vi "Process Message.vi"(8 "error in (no error)":errorcluster, 9 "Error From Read":errorcluster, 10 "Message":string, 11 "tWorkerTCPConnection in":refnum<class "tWorkerTCPConnection.lvclass">) -> (0 "error out":errorcluster, 3 "tWorkerTCPConnection out":refnum<class "tWorkerTCPConnection.lvclass">)   [LabVIEW 2014, in "tWorkerTCPConnection.lvlib" / "tWorkerTCPConnection.lvclass"]
uses:
  tWorkerTCPConnection.lvclass
  tWorkerTCPConnection.lvclass/tWorkerTCPConnection.ctl
  tWorkerCommandRunner/msgs/Run VI Msg/Run VI.lvclass/Run VI.ctl
  <vilib>/ActorFramework/Message Enqueuer/Message Enqueuer.lvclass/Message Enqueuer.ctl
  BSON/tBSONDocument/tBSONDocument.lvclass
  <vilib>/ActorFramework/Actor/Actor.lvclass/Actor.ctl
  tWorkerController/msgs/TCP Connection Lost Msg/TCP Connection Lost Msg.lvclass/TCP Connection Lost Msg.ctl
  <vilib>/ActorFramework/Message Enqueuer/Enqueue.vi
  <vilib>/ActorFramework/Message Enqueuer/Init from Existing Queue.vi
  BSON/tBSONDocument/getStringValue.vi
  BSON/tBSONDocument/getI32Value.vi
  BSON/tBSONDocument/getBooleanValue.vi
  BSON/tBSONDocument/getString[]Value.vi
  BSON/tBSONDocument/getDocumentValue.vi
  <vilib>/ActorFramework/Message Priority Queue/Priority Enqueue.vi
  tWorkerCommandRunner/msgs/Run VI Msg/Run VI.lvclass
  <vilib>/ActorFramework/Message Enqueuer/Message Enqueuer.lvclass
  tWorkerController/msgs/TCP Connection Lost Msg/TCP Connection Lost Msg.lvclass
  <vilib>/ActorFramework/Stop Msg/Stop Msg.lvclass
  <vilib>/ActorFramework/Actor/Actor.lvclass
  tWorkerController/msgs/TCP Command Received Msg/TCP Command Received Msg.lvclass
  tWorkerCommandRunner/msgs/Describe Error Msg/Describe Error Msg.lvclass
  tWorkerCommandRunner/msgs/Set Controls Msg/Set Controls.lvclass
  tWorkerCommandRunner/msgs/Get Indicators Msg/Get Indicators.lvclass
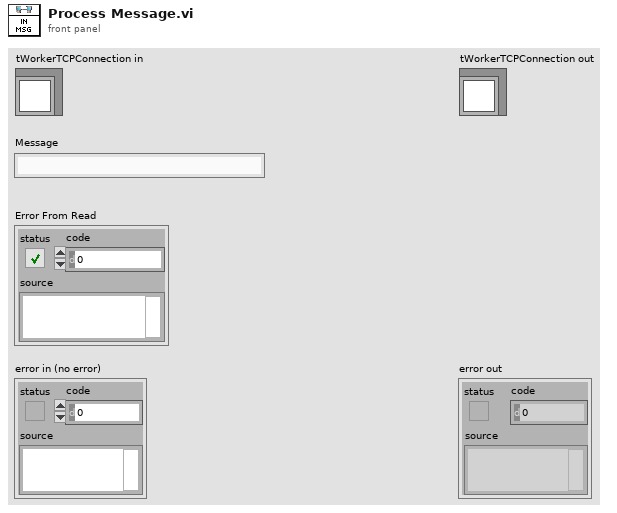
[diagram p1: front panel]
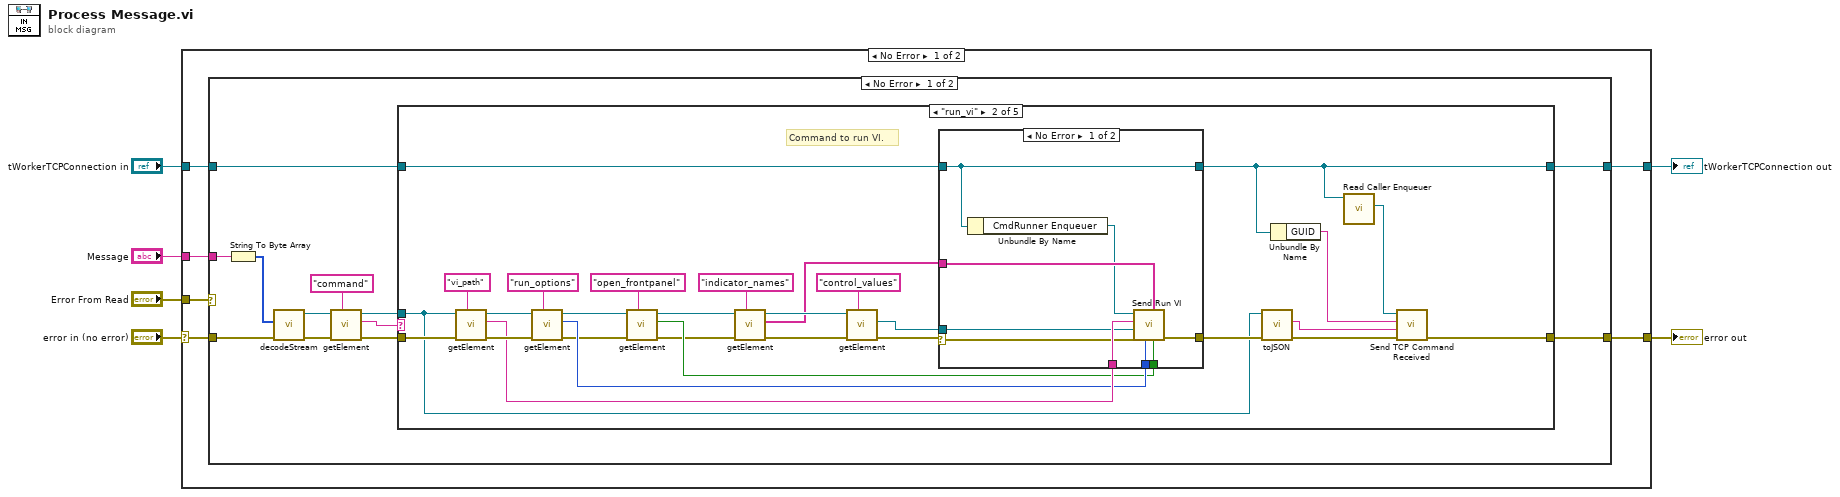
[diagram p0: block diagram]
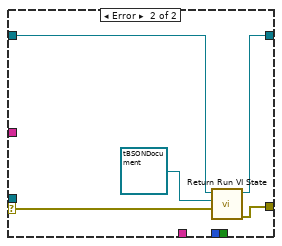
[diagram p3: hidden frame]
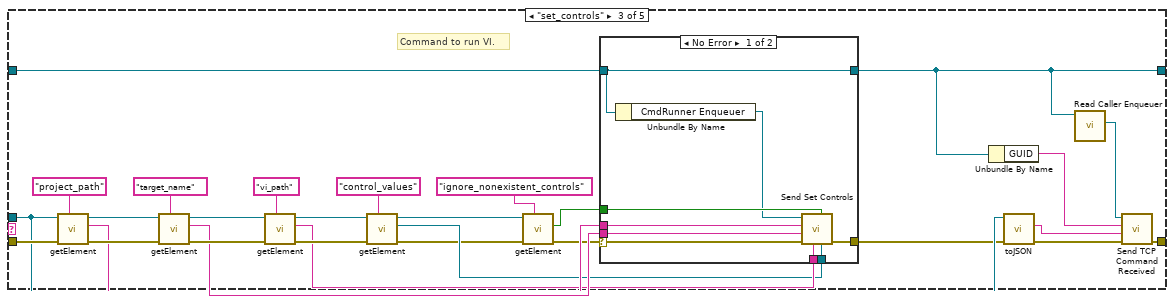
[diagram p4: hidden frame]
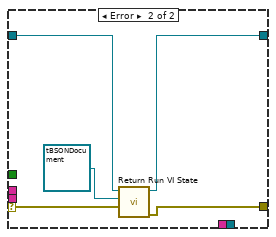
[diagram p5: hidden frame]
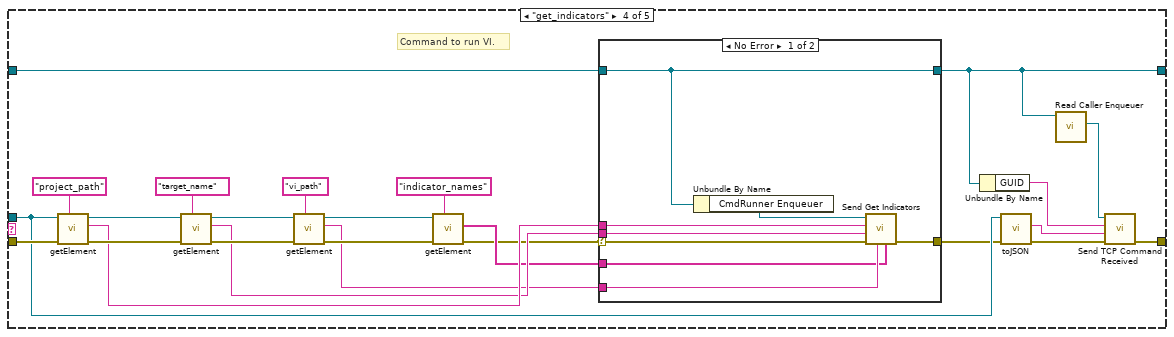
[diagram p6: hidden frame]
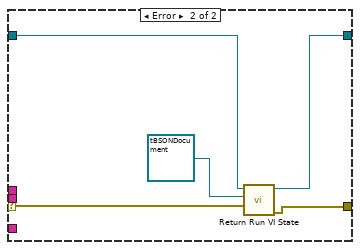
[diagram p7: hidden frame]
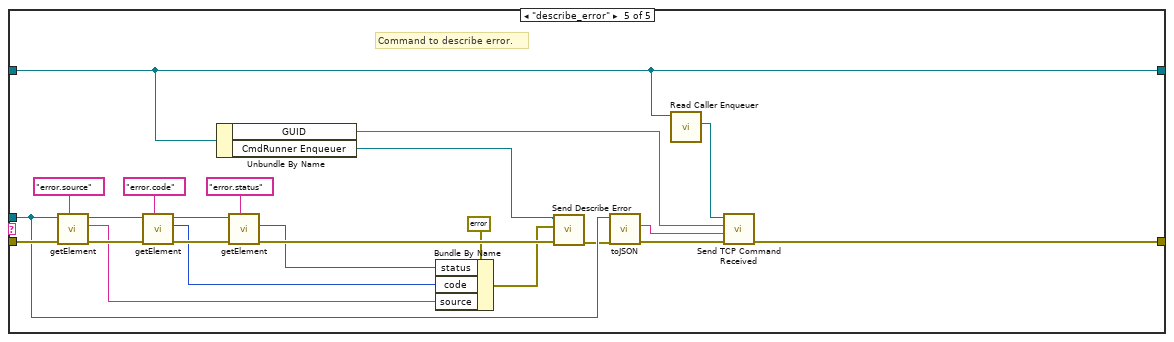
[diagram p8: hidden frame]
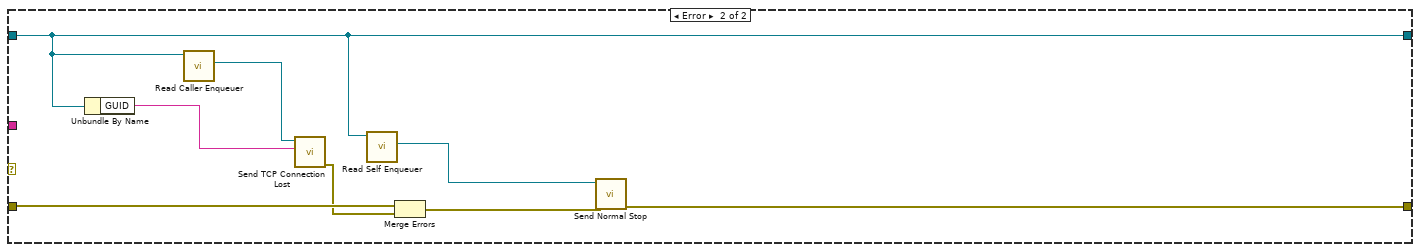
[diagram p9: hidden frame]
diagram:
  n1 = case shown="No Error" "error in (no error)" {
    selector: "error in (no error)" -> [w10 w183]
    tunnel: [w7 w183] -> w5
    tunnel: [w8 w182] -> w3
    tunnel: "tWorkerTCPConnection in" -> [w12 w182]
    tunnel: "Message" -> [w11 _]
    tunnel: "Error From Read" -> [w9 _]
    frame No Error {
      n2 = case shown="No Error" w9 {
        tunnel: w12 -> [w24 w174]
        tunnel: w11 -> [w22 _]
        tunnel: w10 -> [w23 w179]
        tunnel: [w20 w174] -> w8
        tunnel: [w19 w176] -> w7
        frame No Error {
          n3 = String To Byte Array(string=w22) -> (unsigned byte array=w21:u8[])
          n4 = call "decodeStream.vi"("error in (no error)"=w23, "Byte Data In"=w21) -> ("error out"=w17:errorcluster, "tBSONDocument out"=w18:refnum<class "tBSONDocument.lvclass">)  [unwired: 6 in, 2 out]
          n5 = call-poly "getElement.vi"("Name"="command", "error in (no error)"=w17, "tBSONDocument in"=w18) -> ("error out"=w15:errorcluster, "Value"=w13:string, "tBSONDocument out"=w16:refnum<class "tBSONDocument.lvclass">)  [unwired: 6 in]
          n6 = case shown="\"run_vi\"" w13 {
            tunnel: w24 -> [w25 w29 w72 w116 w168]
            tunnel: w16 -> [_ w42 w89 w128 w163]
            tunnel: w15 -> [w26 w50 w93 w132 w169]
            tunnel: [w25 w28 w71 w113 w168] -> w20
            tunnel: [w26 w46 w92 w131 w167] -> w19
            frame Default {
              # "Invalid Command"
            }
            frame "run_vi" {
              # "Command to run VI."
              n7 = call-poly "getElement.vi"("Name"="vi_path", "error in (no error)"=w50, "tBSONDocument in"=w42) -> ("error out"=w55:errorcluster, "Value"=w49:string, "tBSONDocument out"=w54:refnum<class "tBSONDocument.lvclass">)  [unwired: 6 in]
              n8 = call-poly "getElement.vi"("Name"="run_options", "error in (no error)"=w55, "tBSONDocument in"=w54) -> ("error out"=w40:errorcluster, "Value"=w47:i32, "tBSONDocument out"=w39:refnum<class "tBSONDocument.lvclass">)  [unwired: 6 in]
              n9 = call-poly "getElement.vi"("Name"="open_frontpanel", "error in (no error)"=w40, "tBSONDocument in"=w39) -> ("error out"=w34:errorcluster, "Value"=w37:bool, "tBSONDocument out"=w35:refnum<class "tBSONDocument.lvclass">)  [unwired: 6 in]
              n10 = call-poly "getElement.vi"("Name"="indicator_names", "error in (no error)"=w34, "tBSONDocument in"=w35) -> ("error out"=w32:errorcluster, "Value"=w31:string[], "tBSONDocument out"=w33:refnum<class "tBSONDocument.lvclass">)  [unwired: 6 in]
              n11 = call-poly "getElement.vi"("Name"="control_values", "error in (no error)"=w32, "tBSONDocument in"=w33) -> ("error out"=w30:errorcluster, "Value"=w48:refnum<class "tBSONDocument.lvclass">)  [unwired: 6 in, 1 out]
              n12 = case shown="No Error" w30 {
                selector: w30 -> [w58 w69]
                tunnel: w49 -> [w64 _]
                tunnel: w48 -> [w63 _]
                tunnel: w47 -> [w62 _]
                tunnel: [w61 w66] -> w44
                tunnel: w37 -> [w60 _]
                tunnel: w31 -> [w59 _]
                tunnel: w29 -> [w57 w68]
                tunnel: [w57 w67] -> w28
                frame No Error {
                  n13 = Unbundle By Name(w57) -> ("CmdRunner Enqueuer"=w56:refnum<class "Message Enqueuer.lvclass">)
                  n14 = call "Send Run VI.vi"("Open Front Panel"=w60, "Indicator Names"=w59, "Run Options"=w62, "error in (no error)"=w58, "VI Control Values"=w63, "VI Path"=w64, "Message Enqueuer"=w56) -> ("error out"=w61:errorcluster)  [unwired: 3 in, 1 out]
                }
                frame Error {
                  n15 = call "Return Run VI State.vi"("Error From Run VI"=w69, "Indicators"=refnum<class "tBSONDocument.lvclass"> refnum, "tWorkerTCPConnection in"=w68) -> ("error out"=w66:errorcluster, "tWorkerTCPConnection out"=w67:refnum<class "tWorkerTCPConnection.lvclass">)  [unwired: 7 in]
                }
              }
              n16 = call-dynamic "toJSON.vi"("error in (no error)"=w44, "tBSONDocument in"=w42) -> ("error out"=w43:errorcluster, "JSON"=w41:string)  [unwired: 7 in, 1 out]
              n17 = Unbundle By Name(w28) -> ("GUID"=w27:string)
              n18 = call <vilib>:"Read Caller Enqueuer.vi"("Actor"=w28) -> ("Caller Enqueuer"=w45:refnum<class "Message Enqueuer.lvclass">)  [unwired: 10 in]
              n19 = call "Send TCP Command Received.vi"("error in (no error)"=w43, "Message"=w41, "GUID"=w27, "Message Enqueuer"=w45) -> ("error out"=w46:errorcluster)  [unwired: 6 in, 1 out]
            }
            frame "set_controls" {
              # "Command to run VI."
              n20 = call-poly "getElement.vi"("Name"="project_path", "error in (no error)"=w93, "tBSONDocument in"=w89) -> ("error out"=w98:errorcluster, "Value"=w82:string, "tBSONDocument out"=w97:refnum<class "tBSONDocument.lvclass">)  [unwired: 6 in]
              n21 = call-poly "getElement.vi"("Name"="target_name", "error in (no error)"=w98, "tBSONDocument in"=w97) -> ("error out"=w87:errorcluster, "Value"=w81:string, "tBSONDocument out"=w86:refnum<class "tBSONDocument.lvclass">)  [unwired: 6 in]
              n22 = call-poly "getElement.vi"("Name"="vi_path", "error in (no error)"=w87, "tBSONDocument in"=w86) -> ("error out"=w84:errorcluster, "Value"=w80:string, "tBSONDocument out"=w85:refnum<class "tBSONDocument.lvclass">)  [unwired: 6 in]
              n23 = call-poly "getElement.vi"("Name"="control_values", "error in (no error)"=w84, "tBSONDocument in"=w85) -> ("error out"=w76:errorcluster, "Value"=w79:refnum<class "tBSONDocument.lvclass">, "tBSONDocument out"=w77:refnum<class "tBSONDocument.lvclass">)  [unwired: 6 in]
              n24 = call-poly "getElement.vi"("Name"="ignore_nonexistent_controls", "error in (no error)"=w76, "tBSONDocument in"=w77) -> ("error out"=w73:errorcluster, "Value"=w74:bool)  [unwired: 6 in, 1 out]
              n25 = case shown="No Error" w73 {
                selector: w73 -> [w101 w112]
                tunnel: w82 -> [w107 _]
                tunnel: w81 -> [w106 _]
                tunnel: w80 -> [w105 _]
                tunnel: w79 -> [w104 _]
                tunnel: [w103 w109] -> w78
                tunnel: w74 -> [w102 _]
                tunnel: w72 -> [w99 w111]
                tunnel: [w99 w110] -> w71
                frame No Error {
                  n26 = Unbundle By Name(w99) -> ("CmdRunner Enqueuer"=w100:refnum<class "Message Enqueuer.lvclass">)
                  n27 = call "Send Set Controls.vi"("VI Control Values"=w104, "Ignore Non-existent Controls"=w102, "VI Path"=w105, "error in (no error)"=w101, "Target Name"=w106, "Project Path"=w107, "Message Enqueuer"=w100) -> ("error out"=w103:errorcluster)  [unwired: 3 in, 1 out]
                }
                frame Error {
                  n28 = call "Return Run VI State.vi"("Error From Run VI"=w112, "Indicators"=refnum<class "tBSONDocument.lvclass"> refnum, "tWorkerTCPConnection in"=w111) -> ("error out"=w109:errorcluster, "tWorkerTCPConnection out"=w110:refnum<class "tWorkerTCPConnection.lvclass">)  [unwired: 7 in]
                }
              }
              n29 = Unbundle By Name(w71) -> ("GUID"=w70:string)
              n30 = call-dynamic "toJSON.vi"("error in (no error)"=w78, "tBSONDocument in"=w89) -> ("error out"=w90:errorcluster, "JSON"=w88:string)  [unwired: 7 in, 1 out]
              n31 = call <vilib>:"Read Caller Enqueuer.vi"("Actor"=w71) -> ("Caller Enqueuer"=w91:refnum<class "Message Enqueuer.lvclass">)  [unwired: 10 in]
              n32 = call "Send TCP Command Received.vi"("error in (no error)"=w90, "Message"=w88, "GUID"=w70, "Message Enqueuer"=w91) -> ("error out"=w92:errorcluster)  [unwired: 6 in, 1 out]
            }
            frame "get_indicators" {
              # "Command to run VI."
              n33 = call-poly "getElement.vi"("Name"="project_path", "error in (no error)"=w132, "tBSONDocument in"=w128) -> ("error out"=w137:errorcluster, "Value"=w121:string, "tBSONDocument out"=w136:refnum<class "tBSONDocument.lvclass">)  [unwired: 6 in]
              n34 = call-poly "getElement.vi"("Name"="target_name", "error in (no error)"=w137, "tBSONDocument in"=w136) -> ("error out"=w126:errorcluster, "Value"=w120:string, "tBSONDocument out"=w125:refnum<class "tBSONDocument.lvclass">)  [unwired: 6 in]
              n35 = call-poly "getElement.vi"("Name"="vi_path", "error in (no error)"=w126, "tBSONDocument in"=w125) -> ("error out"=w123:errorcluster, "Value"=w118:string, "tBSONDocument out"=w124:refnum<class "tBSONDocument.lvclass">)  [unwired: 6 in]
              n36 = call-poly "getElement.vi"("Name"="indicator_names", "error in (no error)"=w123, "tBSONDocument in"=w124) -> ("error out"=w114:errorcluster, "Value"=w117:string[])  [unwired: 6 in, 1 out]
              n37 = case shown="No Error" w114 {
                selector: w114 -> [w139 w150]
                tunnel: w121 -> [w144 _]
                tunnel: w120 -> [w143 _]
                tunnel: [w142 w149] -> w119
                tunnel: w118 -> [w141 _]
                tunnel: w117 -> [w140 _]
                tunnel: w116 -> [w138 w148]
                tunnel: [w138 w147] -> w113
                frame No Error {
                  n38 = Unbundle By Name(w138) -> ("CmdRunner Enqueuer"=w145:refnum<class "Message Enqueuer.lvclass">)
                  n39 = call "Send Get Indicators.vi"("Indicator Names"=w140, "VI Path"=w141, "error in (no error)"=w139, "Target Name"=w143, "Project Path"=w144, "Message Enqueuer"=w145) -> ("error out"=w142:errorcluster)  [unwired: 4 in, 1 out]
                }
                frame Error {
                  n40 = call "Return Run VI State.vi"("Error From Run VI"=w150, "Indicators"=refnum<class "tBSONDocument.lvclass"> refnum, "tWorkerTCPConnection in"=w148) -> ("error out"=w149:errorcluster, "tWorkerTCPConnection out"=w147:refnum<class "tWorkerTCPConnection.lvclass">)  [unwired: 7 in]
                }
              }
              n41 = Unbundle By Name(w113) -> ("GUID"=w115:string)
              n42 = call-dynamic "toJSON.vi"("error in (no error)"=w119, "tBSONDocument in"=w128) -> ("error out"=w129:errorcluster, "JSON"=w127:string)  [unwired: 7 in, 1 out]
              n43 = call <vilib>:"Read Caller Enqueuer.vi"("Actor"=w113) -> ("Caller Enqueuer"=w130:refnum<class "Message Enqueuer.lvclass">)  [unwired: 10 in]
              n44 = call "Send TCP Command Received.vi"("error in (no error)"=w129, "Message"=w127, "GUID"=w115, "Message Enqueuer"=w130) -> ("error out"=w131:errorcluster)  [unwired: 6 in, 1 out]
            }
            frame "describe_error" {
              # "Command to describe error."
              n45 = call-poly "getElement.vi"("Name"="error.source", "error in (no error)"=w169, "tBSONDocument in"=w163) -> ("error out"=w173:errorcluster, "Value"=w152:string, "tBSONDocument out"=w172:refnum<class "tBSONDocument.lvclass">)  [unwired: 6 in]
              n46 = call-poly "getElement.vi"("Name"="error.code", "error in (no error)"=w173, "tBSONDocument in"=w172) -> ("error out"=w161:errorcluster, "Value"=w153:i32, "tBSONDocument out"=w160:refnum<class "tBSONDocument.lvclass">)  [unwired: 6 in]
              n47 = Unbundle By Name(w168) -> ("GUID"=w165:string, "CmdRunner Enqueuer"=w158:refnum<class "Message Enqueuer.lvclass">)
              n48 = call-poly "getElement.vi"("Name"="error.status", "error in (no error)"=w161, "tBSONDocument in"=w160) -> ("error out"=w156:errorcluster, "Value"=w154:bool)  [unwired: 6 in, 1 out]
              n49 = Bundle By Name(cluster=errorcluster {"status"=FALSE, "code"=0, "source"=""} ("error constant"), "status"=w154, "code"=w153, "source"=w152) -> (w151:errorcluster)
              n50 = call "Send Describe Error.vi"("error in (no error)"=w156, "error"=w151, "Message Enqueuer"=w158) -> ("error out"=w157:errorcluster)  [unwired: 7 in, 1 out]
              n51 = call-dynamic "toJSON.vi"("error in (no error)"=w157, "tBSONDocument in"=w163) -> ("error out"=w164:errorcluster, "JSON"=w162:string)  [unwired: 7 in, 1 out]
              n52 = call <vilib>:"Read Caller Enqueuer.vi"("Actor"=w168) -> ("Caller Enqueuer"=w166:refnum<class "Message Enqueuer.lvclass">)  [unwired: 10 in]
              n53 = call "Send TCP Command Received.vi"("error in (no error)"=w164, "Message"=w162, "GUID"=w165, "Message Enqueuer"=w166) -> ("error out"=w167:errorcluster)  [unwired: 6 in, 1 out]
            }
          }
        }
        frame Error {
          n54 = Unbundle By Name(w174) -> ("GUID"=w180:string)
          n55 = call <vilib>:"Read Caller Enqueuer.vi"("Actor"=w174) -> ("Caller Enqueuer"=w181:refnum<class "Message Enqueuer.lvclass">)  [unwired: 10 in]
          n56 = call "Send TCP Connection Lost.vi"("Connection GUID"=w180, "Message Enqueuer"=w181) -> ("error out"=w178:errorcluster)  [unwired: 8 in, 1 out]
          n57 = call <vilib>:"Read Self Enqueuer.vi"("Actor"=w174) -> ("Self Enqueuer"=w175:refnum<class "Message Enqueuer.lvclass">)  [unwired: 10 in]
          n58 = Merge Errors(w179, w178) -> (w177:errorcluster)
          n59 = call <vilib>:"Send Normal Stop.vi"("error in (no error)"=w177, "Message Enqueuer"=w175) -> ("error out"=w176:errorcluster)  [unwired: 9 in]
        }
      }
    }
    frame Error {
    }
  }
  "error out" <- w5
  "tWorkerTCPConnection out" <- w3
